vi "MRC Ds Comms Control Set Has User Code.vi"(8 "error in (no error)":errorcluster, 11 "hasUserCode":u8) -> (0 "error out":errorcluster)   [LabVIEW 2026, in "MrcLib.lvlib"]
doc: "MRC_Status MRC_CALLCONV MRC_DsCommsControl_SetHasUserCode(MRC_Bool hasUserCode);"
uses:
  MrcLib.lvlib
  MrcLib.dll
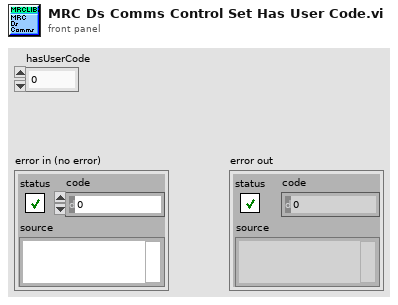
[diagram p1: front panel]
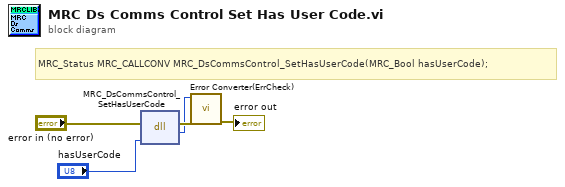
[diagram p0: block diagram]
diagram:
  # "MRC_Status MRC_CALLCONV MRC_DsCommsControl_SetHasUserCode(MRC_Bool hasUserCode);"
  n1 = dll-call lib="MrcLib.*" fn="MRC_DsCommsControl_SetHasUserCode"(error in="error in (no error)", "hasUserCode"="hasUserCode") -> (error out=w3:errorcluster, "return type"=w1:i32)  [unwired: 3 in, 1 out]
  n2 = call <vilib>:"Error Converter(ErrCheck).vi"("error in (no error)"=w3, "status"=w1) -> ("error out"=→"error out":errorcluster)  [unwired: 9 in]
